vi "BMU诊断标定.vi"(8 "CAN端口":u16(ring), 9 "设备索引号":u16(ring), 10 "CAN卡类型":u32(ring)=21) -> ()   [LabVIEW 2013] (continued)
                                n3887 = property class="Str"(reference=w5555, "Value"="" ("值")) -> ()  [unwired: 1 in, 2 out]
                                }
                                frame "校正时钟" {
                                n3888 = control-ref of="系统时钟"() -> (w5557:refnum<vi>)
                                n3889 = property class="Str"(reference=w5557, "Value"="" ("值")) -> ()  [unwired: 1 in, 2 out]
                                }
                                frame "车牌号" {
                                n3890 = control-ref of="车架(牌)号"() -> (w5559:refnum<vi>)
                                n3891 = property class="Str"(reference=w5559, "Value"="" ("值")) -> ()  [unwired: 1 in, 2 out]
                                }
                                frame "SOH" {
                                n3892 = control-ref of="SOH(%)"() -> (w5562:refnum<vi>)
                                n3893 = property class="DigNum (严格)"(reference=w5562, "Value"=0.0 ("值")) -> ()  [unwired: 1 in, 2 out]
                                }
                                frame "一级故障阀值" {
                                n3894 = local write "一级故障"(T10 {"总电压过高"=0.0, "整组电压不均衡"=0.0, "SOC过高"=0.0, "单体电压过高"=0.0, "总电压过低"=0.0, "温度过高"=0.0, "温度过低"=0.0, "单组电压不均衡"=0.0, "整组温度不均衡"=0.0, "单组温度不均衡"=0.0, "单体电压过低"=0.0, "充电电流过高"=0.0, "放电电流过高"=0.0, "SOC过低"=0.0, "内阻过大"=0.0, "极柱温度过高"=0.0, "SOH过低"=0.0} ("一级故障")) -> ()
                                }
                                frame "二级故障阀值" {
                                n3895 = local write "一级故障 2"(T10 {"总电压过高"=0.0, "整组电压不均衡"=0.0, "SOC过高"=0.0, "单体电压过高"=0.0, "总电压过低"=0.0, "温度过高"=0.0, "温度过低"=0.0, "单组电压不均衡"=0.0, "整组温度不均衡"=0.0, "单组温度不均衡"=0.0, "单体电压过低"=0.0, "充电电流过高"=0.0, "放电电流过高"=0.0, "SOC过低"=0.0, "内阻过大"=0.0, "极柱温度过高"=0.0, "SOH过低"=0.0} ("一级故障")) -> ()
                                }
                                frame "三级故障阀值" {
                                n3896 = local write "一级故障 3"(T10 {"总电压过高"=0.0, "整组电压不均衡"=0.0, "SOC过高"=0.0, "单体电压过高"=0.0, "总电压过低"=0.0, "温度过高"=0.0, "温度过低"=0.0, "单组电压不均衡"=0.0, "整组温度不均衡"=0.0, "单组温度不均衡"=0.0, "单体电压过低"=0.0, "充电电流过高"=0.0, "放电电流过高"=0.0, "SOC过低"=0.0, "内阻过大"=0.0, "极柱温度过高"=0.0, "SOH过低"=0.0} ("一级故障")) -> ()
                                }
                                frame "加热控制参数" {
                                n3897 = local write "加热控制参数"(T11 {"风机开启温度"=0.0, "风机关闭温度"=0.0, "加热开启温度"=0.0, "加热关闭温度"=0.0, "风机开启温差"=0.0, "风机关闭温差"=0.0, "加热关闭温差"=0.0} ("加热控制参数")) -> ()
                                }
                                frame "充电控制参数" {
                                n3898 = local write "一级故障 5"(T12 {"最大允许单体电压"=0.0, "最大允许总电压"=0.0, "最小允许单体电压"=0.0, "最大允许充电电流"=0.0, "最小允许充电电流"=0.0, "最大允许充电温度"=0.0, "最小允许充电温度"=0.0, "电流步长"=0.0} ("一级故障 5")) -> ()
                                }
                                frame "电池信息1" {
                                w5568 = ""
                                w5569 = 0.0 ("电池串联")
                                n3899 = local read "电池信息"() -> (w5571:T13)
                                n3900 = Bundle By Name(cluster=w5571, "电池串联"=w5569, "电池并联"=w5569, "电池包额定容量"=w5569, "电池包额定能量(kWh)"=w5569, "电池包额定总电压"=w5569, "实际容量"=w5569, "电池厂家"=w5568, "电池类型"=w5568, "电池生产日期"=w5568) -> (w5570:T13)
                                n3901 = local write "电池信息"(w5570) -> ()
                                }
                                frame "电池包组号" {
                                n3902 = local read "电池信息"() -> (w5574:T13)
                                n3903 = Bundle By Name(cluster=w5574, "电池包组号"="") -> (w5573:T13)
                                n3904 = local write "电池信息"(w5573) -> ()
                                }
                                frame "充放电安时" {
                                w5575 = 0.0 ("累计充电总安时")
                                n3905 = local read "电池信息"() -> (w5577:T13)
                                n3906 = Bundle By Name(cluster=w5577, "累计充电总安时"=w5575, "累计放电总安时"=w5575) -> (w5576:T13)
                                n3907 = local write "电池信息"(w5576) -> ()
                                }
                                frame "电池充放电次数" {
                                w5578 = 0.0 ("累计充电总安时")
                                n3908 = local read "电池信息"() -> (w5580:T13)
                                n3909 = Bundle By Name(cluster=w5580, "电池充满次数"=w5578, "电池放空次数"=w5578, "电池充电次数"=w5578) -> (w5579:T13)
                                n3910 = local write "电池信息"(w5579) -> ()
                                }
                                }
                              }
                              frame "从板" {
                                n3911 = case shown="\"温度起始值\"" w5581 {
                                frame "假", Default {
                                }
                                frame "电压起始值" {
                                n3912 = for {
                                N: 1 -> [_]
                                tunnel: [""] -> w5586 mode=indexing
                                }
                                n3913 = control-ref of="项目信息 2"() -> (w5582:refnum<vi>)
                                n3914 = call "表格数据输入-8.6.vi"("行数"=u32 0, "列数"=u32 1, "字符串数组"=w5586, "表格引用"=w5582) -> ()  [unwired: 8 in]
                                }
                                frame "通道电压个数" {
                                n3915 = for {
                                N: 5 -> [_]
                                tunnel: [""] -> w5592 mode=indexing
                                }
                                n3916 = control-ref of="项目信息 2"() -> (w5588:refnum<vi>)
                                n3917 = call "表格数据输入-8.6.vi"("行数"=u32 22, "列数"=u32 1, "字符串数组"=w5592, "表格引用"=w5588) -> ()  [unwired: 8 in]
                                }
                                frame "保险位置" {
                                n3918 = for {
                                N: 10 -> [_]
                                tunnel: [""] -> w5598 mode=indexing
                                }
                                n3919 = control-ref of="项目信息 2"() -> (w5594:refnum<vi>)
                                n3920 = call "表格数据输入-8.6.vi"("行数"=u32 2, "列数"=u32 1, "字符串数组"=w5598, "表格引用"=w5594) -> ()  [unwired: 8 in]
                                }
                                frame "温度起始值" {
                                n3921 = for {
                                N: 1 -> [_]
                                tunnel: [""] -> w5604 mode=indexing
                                }
                                n3922 = control-ref of="项目信息 2"() -> (w5600:refnum<vi>)
                                n3923 = call "表格数据输入-8.6.vi"("行数"=u32 1, "列数"=u32 1, "字符串数组"=w5604, "表格引用"=w5600) -> ()  [unwired: 8 in]
                                }
                                frame "加热控制参数" {
                                n3924 = local write "加热控制参数"(T11 {"风机开启温度"=0.0, "风机关闭温度"=0.0, "加热开启温度"=0.0, "加热关闭温度"=0.0, "风机开启温差"=0.0, "风机关闭温差"=0.0, "加热关闭温差"=0.0} ("加热控制参数")) -> ()
                                }
                                frame "一级故障阀值" {
                                n3925 = local write "一级故障 6"(T15 {"电压过高"=0.0, "电压过低"=0.0, "温度过高"=0.0, "温度过低"=0.0, "电压不均衡(V)"=0.0, "温度不均衡"=0.0, "SOC过低"=0.0} ("一级故障 6")) -> ()
                                }
                                frame "二级故障阀值" {
                                n3926 = local write "一级故障 7"(T15 {"电压过高"=0.0, "电压过低"=0.0, "温度过高"=0.0, "温度过低"=0.0, "电压不均衡(V)"=0.0, "温度不均衡"=0.0, "SOC过低"=0.0} ("一级故障 7")) -> ()
                                }
                                frame "三级故障阀值" {
                                n3927 = local write "一级故障 8"(T15 {"电压过高"=0.0, "电压过低"=0.0, "温度过高"=0.0, "温度过低"=0.0, "电压不均衡(V)"=0.0, "温度不均衡"=0.0, "SOC过低"=0.0} ("一级故障 7")) -> ()
                                }
                                frame "均衡参数" {
                                n3928 = local write "均衡参数"(T17 {"充电结束电压(90%)"=0.0, "充电结束电压(91%)"=0.0, "充电结束电压(92%)"=0.0, "充电结束电压(93%)"=0.0, "充电结束电压(94%)"=0.0, "均衡计算-电压高阀值1级"=0.0, "均衡计算-电压高阀值2级"=0.0, "均衡计算-电压低阀值1级"=0.0, "均衡计算-电压低阀值2级"=0.0, "均衡计算-最低电压阀值"=0.0, "均衡停止-最低电压阀值"=0.0, "均衡计算-电压极差阀值"=0.0, "充电结束电压(95%)"=0.0, "充电结束电压(96%)"=0.0, "充电结束电压(97%)"=0.0, "充电结束电压(98%)"=0.0, "充电结束电压(99%)"=0.0, "充电结束电压(100%)"=0.0} ("均衡参数")) -> ()
                                }
                                frame "均衡阀值" {
                                w5611 = sgl 0.0 ("均衡计算-电压高阀值1级")
                                n3929 = local read "均衡参数"() -> (w5612:T17)
                                n3930 = Bundle By Name(cluster=w5612, "均衡计算-电压高阀值1级"=w5611, "均衡计算-电压高阀值2级"=w5611, "均衡计算-电压低阀值1级"=w5611, "均衡计算-电压低阀值2级"=w5611, "均衡计算-最低电压阀值"=w5611, "均衡停止-最低电压阀值"=w5611, "均衡计算-电压极差阀值"=w5611) -> (w5613:T17)
                                n3931 = local write "均衡参数"(w5613) -> ()
                                }
                                frame "充电结束电压" {
                                w5614 = sgl 0.0 ("均衡计算-电压高阀值1级")
                                n3932 = local read "均衡参数"() -> (w5615:T17)
                                n3933 = Bundle By Name(cluster=w5615, "充电结束电压(90%)"=w5614, "充电结束电压(91%)"=w5614, "充电结束电压(92%)"=w5614, "充电结束电压(93%)"=w5614, "充电结束电压(94%)"=w5614, "充电结束电压(95%)"=w5614, "充电结束电压(96%)"=w5614, "充电结束电压(97%)"=w5614, "充电结束电压(98%)"=w5614, "充电结束电压(99%)"=w5614, "充电结束电压(100%)"=w5614) -> (w5616:T17)
                                n3934 = local write "均衡参数"(w5616) -> ()
                                }
                                }
                              }
                            }
                          }
                          frame #1 {
                            w5617 = FALSE ("流控帧")
                            w5618 = TRUE ("流控帧 2")
                            n3935 = global write "EV05全局变量1.vi" "写入超时"(w5617) -> ()
                            n3936 = global write "EV05全局变量1.vi" "流控帧"(w5617) -> ()
                            n3937 = local write "写?"(w5617) -> ()
                            n3938 = local write "消除"(w5618) -> ()
                            n3939 = local write "控制1"(w5618) -> ()
                            n3940 = global write "EV05全局变量1.vi" "流控帧 2"(w5618) -> ()
                          }
                          frame #2 {
                            n3941 = Wait Until Next ms Multiple(millisecond multiple=u32 300 ("毫秒倍数")) -> ()  [unwired: 1 out]
                          }
                          frame #3 {
                            n3942 = local read "设备索引号"() -> (w5621:u16)
                            n3943 = local read "CAN卡类型"() -> (w5622:u32)
                            n3944 = local read "CAN端口"() -> (w5620:u16)
                            n3945 = local write "命令序号"(w5625) -> ()
                            n3946 = stacked-sequence {
                              tunnel: w5626 -> [_ w5633]
                              tunnel: w5625 -> [_ w5632]
                              tunnel: w5624 -> [_ w5631]
                              tunnel: w5623 -> [_ w5630]
                              tunnel: w5622 -> [_ w5629]
                              tunnel: w5621 -> [_ w5628]
                              tunnel: w5620 -> [_ w5627]
                              frame #0 {
                              }
                              frame #1 {
                                n3947 = call "多帧发送机制(EV05).vi"("can卡类型"=w5629, "设备索引号"=w5628, "CAN端口"=w5627, "命令"=w5633, "板号"=w5631, "命令序号"=w5632, "输入数据"=w5630) -> ()  [unwired: 1 in, 12 out]
                              }
                            }
                          }
                          frame #4 {
                            n3948 = while {
                              tunnel: [w5638] -> w5635
                              tunnel: [w5637] -> w5634
                              i -> [w5641]
                              stop <- w5638 stop-if-true
                              n3949 = local read "强制终止读写标记"() -> (w5636:bool)
                              n3950 = global read "EV05全局变量1.vi" "写入超时"() -> (w5637:bool)
                              n3951 = Greater Or Equal?(x=w5641, y=20) -> (x >= y?=w5639:bool)
                              n3952 = Compound Arithmetic op=OR(w5636, w5637, w5639) -> (w5638:bool)
                              n3953 = Wait Until Next ms Multiple(millisecond multiple=u32 100 ("毫秒倍数")) -> ()  [unwired: 1 out]
                            }
                          }
                          frame #5 {
                            n3954 = case shown="假" w5650 {
                              tunnel: w5649 -> [w5661 _]
                              tunnel: [w5656 w5673] -> w5648
                              tunnel: w5647 -> [w5655 _]
                              tunnel: w5646 -> [w5654 w5673]
                              tunnel: [w5653 w5672] -> w5643
                              tunnel: w5645 -> [w5652 _]
                              tunnel: w5644 -> [w5651 w5672]
                              frame False {
                                n3955 = local read "重试次数"() -> (w5660:u8)
                                n3956 = Increment(x=w5660) -> (x+1=w5659:u8)
                                n3957 = Greater Or Equal?(x=w5659, y=u8 4) -> (x >= y?=w5658:bool)
                                n3958 = local write "重试次数"(w5659) -> ()
                                n3959 = case shown="真" w5658 {
                                tunnel: w5661 -> [_ w5666]
                                tunnel: [w5663 w5665] -> w5656
                                tunnel: w5655 -> [w5663 _]
                                tunnel: w5654 -> [_ w5665]
                                tunnel: [w5662 w5664] -> w5653
                                tunnel: w5652 -> [w5662 _]
                                tunnel: w5651 -> [_ w5664]
                                frame False {
                                }
                                frame True {
                                n3960 = control-ref of="结果"() -> (w5668:refnum<vi>)
                                n3961 = Concatenate Strings(w5666, "     读取失败" ("字符串")) -> (w5670:string)
                                n3962 = Build Array(w5670) -> (w5667:string[])
                                n3963 = call "表格编辑.vi"("新元素/子数组"=w5667, "活动单元格:单元格背景色"=u32 16740749, "MCListbox引用句柄"=w5668) -> ()  [unwired: 9 out]
                                }
                                }
                              }
                              frame True {
                              }
                            }
                          }
                          frame #6 {
                            n3964 = And(x=w5675, y=w5677) -> (x .and. y?=w5676:bool)
                            n3965 = case shown="真" w5676 {
                              frame False {
                              }
                              frame True {
                                n3966 = local write "强制终止读写标记"(FALSE ("强制停止")) -> ()
                                n3967 = control-ref of="结果"() -> (w5680:refnum<vi>)
                                n3968 = Concatenate Strings("读取完成" ("字符串")) -> (w5682:string)
                                n3969 = Build Array(w5682) -> (w5679:string[])
                                n3970 = call "表格编辑.vi"("新元素/子数组"=w5679, "活动单元格:单元格背景色"=u32 21937, "MCListbox引用句柄"=w5680) -> ()  [unwired: 9 out]
                              }
                            }
                            n3971 = Wait (ms)(milliseconds to wait=u32 50 ("等待时间（毫秒）")) -> ()  [unwired: 1 out]
                          }
                        }
                      }
                    }
                  }
                  n3972 = local read "强制终止读写标记"() -> (w5448:bool)
                  n3973 = Or(x=w5448, y=w5447) -> (x .or. y?=w5445:bool)
                }
              }
            }
            frame #2 {
              n3974 = case shown="假" w5767 {
                tunnel: w5768 -> [w5769 _]
                frame False {
                  n3975 = case shown="\"主板\", 默认" w5769 {
                    frame "主板", Default {
                      n3976 = global read "读配置文件全局.vi" "电池额定实际容量判定"() -> (w5783:bool)
                      n3977 = global read "读配置文件全局.vi" "电池充放电次数判定"() -> (w5772:bool)
                      n3978 = global read "读配置文件全局.vi" "加热控制参数判定"() -> (w5770:bool)
                      n3979 = global read "读配置文件全局.vi" "配置文件版本判定"() -> (w5782:bool)
                      n3980 = global read "读配置文件全局.vi" "充电控制参数判定"() -> (w5776:bool)
                      n3981 = global read "读配置文件全局.vi" "通道电压数判定"() -> (w5788:bool)
                      n3982 = global read "读配置文件全局.vi" "电压起始值判定"() -> (w5787:bool)
                      n3983 = global read "读配置文件全局.vi" "温度起始值判定"() -> (w5785:bool)
                      n3984 = global read "读配置文件全局.vi" "充放电安时判定"() -> (w5774:bool)
                      n3985 = global read "读配置文件全局.vi" "电池包组号判定"() -> (w5773:bool)
                      n3986 = global read "读配置文件全局.vi" "电池信息1判定"() -> (w5775:bool)
                      n3987 = global read "读配置文件全局.vi" "从板个数判定"() -> (w5791:bool)
                      n3988 = global read "读配置文件全局.vi" "产品编号判定"() -> (w5790:bool)
                      n3989 = global read "读配置文件全局.vi" "电压个数判定"() -> (w5789:bool)
                      n3990 = global read "读配置文件全局.vi" "温度个数判定"() -> (w5786:bool)
                      n3991 = global read "读配置文件全局.vi" "保险位置判定"() -> (w5784:bool)
                      n3992 = global read "读配置文件全局.vi" "一级故障判定"() -> (w5779:bool)
                      n3993 = global read "读配置文件全局.vi" "二级故障判定"() -> (w5778:bool)
                      n3994 = global read "读配置文件全局.vi" "三级故障判定"() -> (w5777:bool)
                      n3995 = global read "读配置文件全局.vi" "车牌号判定"() -> (w5781:bool)
                      n3996 = global read "读配置文件全局.vi" "SOH判定"() -> (w5780:bool)
                      n3997 = Build Array(w5791, w5790, w5789, w5788, w5787, w5786, w5785, w5784, w5783, w5782, w5781, w5780, w5779, w5778, w5777, w5776, w5775, w5774, w5773, w5772, w5770) -> (w5771:bool[])
                      n3998 = And Array Elements(Boolean array=w5771) -> (logical AND=w5792:bool)
                      n3999 = disable-structure shown="禁用" {
                        frame Disabled {
                          n4000 = global read "读配置文件全局.vi" "SOC判定"() -> ()  [unwired: 1 out]
                        }
                        frame Enabled {
                        }
                      }
                      n4001 = case shown="假" w5792 {
                        tunnel: w5771 -> [_ w5797]
                        frame True {
                          n4002 = control-ref of="结果"() -> (w5795:refnum<vi>)
                          n4003 = Build Array("全部判定成功!!!!!!!!") -> (w5796:string[])
                          n4004 = call "表格编辑.vi"("新元素/子数组"=w5796, "活动单元格:单元格背景色"=u32 6618880, "MCListbox引用句柄"=w5795) -> ()  [unwired: 9 out]
                        }
                        frame False {
                          n4005 = stacked-sequence {
                            tunnel: w5797 -> [_ w5802]
                            frame #0 {
                              n4006 = control-ref of="结果"() -> (w5800:refnum<vi>)
                              n4007 = Build Array("全部判定失败!!!!!") -> (w5801:string[])
                              n4008 = call "表格编辑.vi"("新元素/子数组"=w5801, "活动单元格:单元格背景色"=u32 16711680, "MCListbox引用句柄"=w5800) -> ()  [unwired: 9 out]
                            }
                            frame #1 {
                              n4009 = for {
                                tunnel: w5802 -> [w5804] mode=indexing
                                i -> [w5803]
                                n4010 = case shown="20" w5803 {
                                tunnel: w5804 -> [w5805 w5810 w5815 w5820 w5825 w5830 w5835 w5840 w5845 w5850 w5855 w5860 w5865 w5870 w5875 w5880 w5885 w5890 w5895 w5900 w5905 _]
                                frame 0 {
                                n4011 = case shown="假" w5805 {
                                frame False {
                                n4012 = control-ref of="结果"() -> (w5808:refnum<vi>)
                                n4013 = Build Array("从板个数判定失败!") -> (w5809:string[])
                                n4014 = call "表格编辑.vi"("新元素/子数组"=w5809, "活动单元格:单元格背景色"=u32 16711680, "MCListbox引用句柄"=w5808) -> ()  [unwired: 9 out]
                                }
                                frame True {
                                }
                                }
                                }
                                frame 1 {
                                n4015 = case shown="假" w5810 {
                                frame False {
                                n4016 = control-ref of="结果"() -> (w5813:refnum<vi>)
                                n4017 = Build Array("产品编号判定失败!") -> (w5814:string[])
                                n4018 = call "表格编辑.vi"("新元素/子数组"=w5814, "活动单元格:单元格背景色"=u32 16711680, "MCListbox引用句柄"=w5813) -> ()  [unwired: 9 out]
                                }
                                frame True {
                                }
                                }
                                }
                                frame 2 {
                                n4019 = case shown="假" w5815 {
                                frame False {
                                n4020 = control-ref of="结果"() -> (w5818:refnum<vi>)
                                n4021 = Build Array("电压个数判定失败!") -> (w5819:string[])
                                n4022 = call "表格编辑.vi"("新元素/子数组"=w5819, "活动单元格:单元格背景色"=u32 16711680, "MCListbox引用句柄"=w5818) -> ()  [unwired: 9 out]
                                }
                                frame True {
                                }
                                }
                                }
                                frame 3 {
                                n4023 = case shown="假" w5820 {
                                frame False {
                                n4024 = control-ref of="结果"() -> (w5823:refnum<vi>)
                                n4025 = Build Array("通道电压数判定失败!") -> (w5824:string[])
                                n4026 = call "表格编辑.vi"("新元素/子数组"=w5824, "活动单元格:单元格背景色"=u32 16711680, "MCListbox引用句柄"=w5823) -> ()  [unwired: 9 out]
                                }
                                frame True {
                                }
                                }
                                }
                                frame 4 {
                                n4027 = case shown="假" w5825 {
                                frame False {
                                n4028 = control-ref of="结果"() -> (w5828:refnum<vi>)
                                n4029 = Build Array("电压起始值判定失败!") -> (w5829:string[])
                                n4030 = call "表格编辑.vi"("新元素/子数组"=w5829, "活动单元格:单元格背景色"=u32 16711680, "MCListbox引用句柄"=w5828) -> ()  [unwired: 9 out]
                                }
                                frame True {
                                }
                                }
                                }
                                frame 5 {
                                n4031 = case shown="假" w5830 {
                                frame False {
                                n4032 = control-ref of="结果"() -> (w5833:refnum<vi>)
                                n4033 = Build Array("温度个数判定失败!") -> (w5834:string[])
                                n4034 = call "表格编辑.vi"("新元素/子数组"=w5834, "活动单元格:单元格背景色"=u32 16711680, "MCListbox引用句柄"=w5833) -> ()  [unwired: 9 out]
                                }
                                frame True {
                                }
                                }
                                }
                                frame 6 {
                                n4035 = case shown="假" w5835 {
                                frame False {
                                n4036 = control-ref of="结果"() -> (w5838:refnum<vi>)
                                n4037 = Build Array("温度起始值判定失败!") -> (w5839:string[])
                                n4038 = call "表格编辑.vi"("新元素/子数组"=w5839, "活动单元格:单元格背景色"=u32 16711680, "MCListbox引用句柄"=w5838) -> ()  [unwired: 9 out]
                                }
                                frame True {
                                }
                                }
                                }
                                frame 7 {
                                n4039 = case shown="假" w5840 {
                                frame False {
                                n4040 = control-ref of="结果"() -> (w5843:refnum<vi>)
                                n4041 = Build Array("保险位置判定失败!") -> (w5844:string[])
                                n4042 = call "表格编辑.vi"("新元素/子数组"=w5844, "活动单元格:单元格背景色"=u32 16711680, "MCListbox引用句柄"=w5843) -> ()  [unwired: 9 out]
                                }
                                frame True {
                                }
                                }
                                }
                                frame 8 {
                                n4043 = case shown="假" w5845 {
                                frame False {
                                n4044 = control-ref of="结果"() -> (w5848:refnum<vi>)
                                n4045 = Build Array("电池额定实际容量判定失败!") -> (w5849:string[])
                                n4046 = call "表格编辑.vi"("新元素/子数组"=w5849, "活动单元格:单元格背景色"=u32 16711680, "MCListbox引用句柄"=w5848) -> ()  [unwired: 9 out]
                                }
                                frame True {
                                }
                                }
                                }
                                frame 9 {
                                n4047 = case shown="假" w5850 {
                                frame False {
                                n4048 = control-ref of="结果"() -> (w5853:refnum<vi>)
                                n4049 = Build Array("配置文件版本判定失败!") -> (w5854:string[])
                                n4050 = call "表格编辑.vi"("新元素/子数组"=w5854, "活动单元格:单元格背景色"=u32 16711680, "MCListbox引用句柄"=w5853) -> ()  [unwired: 9 out]
                                }
                                frame True {
                                }
                                }
                                }
                                frame 10 {
                                n4051 = case shown="假" w5855 {
                                frame False {
                                n4052 = control-ref of="结果"() -> (w5858:refnum<vi>)
                                n4053 = Build Array("车牌号判定失败!") -> (w5859:string[])
                                n4054 = call "表格编辑.vi"("新元素/子数组"=w5859, "活动单元格:单元格背景色"=u32 16711680, "MCListbox引用句柄"=w5858) -> ()  [unwired: 9 out]
                                }
                                frame True {
                                }
                                }
                                }
                                frame 11 {
                                n4055 = case shown="假" w5860 {
                                frame False {
                                n4056 = control-ref of="结果"() -> (w5863:refnum<vi>)
                                n4057 = Build Array("SOH判定失败!") -> (w5864:string[])
                                n4058 = call "表格编辑.vi"("新元素/子数组"=w5864, "活动单元格:单元格背景色"=u32 16711680, "MCListbox引用句柄"=w5863) -> ()  [unwired: 9 out]
                                }
                                frame True {
                                }
                                }
                                }
                                frame 12 {
                                n4059 = case shown="假" w5865 {
                                frame False {
                                n4060 = control-ref of="结果"() -> (w5868:refnum<vi>)
                                n4061 = Build Array("一级故障阀值判定失败!") -> (w5869:string[])
                                n4062 = call "表格编辑.vi"("新元素/子数组"=w5869, "活动单元格:单元格背景色"=u32 16711680, "MCListbox引用句柄"=w5868) -> ()  [unwired: 9 out]
                                }
                                frame True {
                                }
                                }
                                }
                                frame 13 {
                                n4063 = case shown="假" w5870 {
                                frame False {
                                n4064 = control-ref of="结果"() -> (w5873:refnum<vi>)
                                n4065 = Build Array("二级故障阀值判定失败!") -> (w5874:string[])
                                n4066 = call "表格编辑.vi"("新元素/子数组"=w5874, "活动单元格:单元格背景色"=u32 16711680, "MCListbox引用句柄"=w5873) -> ()  [unwired: 9 out]
                                }
                                frame True {
                                }
                                }
                                }
                                frame 14 {
                                n4067 = case shown="假" w5875 {
                                frame False {
                                n4068 = control-ref of="结果"() -> (w5878:refnum<vi>)
                                n4069 = Build Array("三级故障阀值判定失败!") -> (w5879:string[])
                                n4070 = call "表格编辑.vi"("新元素/子数组"=w5879, "活动单元格:单元格背景色"=u32 16711680, "MCListbox引用句柄"=w5878) -> ()  [unwired: 9 out]
                                }
                                frame True {
                                }
                                }
                                }
                                frame 15 {
                                n4071 = case shown="假" w5880 {
                                frame False {
                                n4072 = control-ref of="结果"() -> (w5883:refnum<vi>)
                                n4073 = Build Array("充电控制参数判定失败!") -> (w5884:string[])
                                n4074 = call "表格编辑.vi"("新元素/子数组"=w5884, "活动单元格:单元格背景色"=u32 16711680, "MCListbox引用句柄"=w5883) -> ()  [unwired: 9 out]
                                }
                                frame True {
                                }
                                }
                                }
                                frame 16 {
                                n4075 = case shown="假" w5885 {
                                frame False {
                                n4076 = control-ref of="结果"() -> (w5888:refnum<vi>)
                                n4077 = Build Array("电池信息1判定失败!") -> (w5889:string[])
                                n4078 = call "表格编辑.vi"("新元素/子数组"=w5889, "活动单元格:单元格背景色"=u32 16711680, "MCListbox引用句柄"=w5888) -> ()  [unwired: 9 out]
                                }
                                frame True {
                                }
                                }
                                }
                                frame 17 {
                                n4079 = case shown="假" w5890 {
                                frame False {
                                n4080 = control-ref of="结果"() -> (w5893:refnum<vi>)
                                n4081 = Build Array("充放电安时判定失败!") -> (w5894:string[])
                                n4082 = call "表格编辑.vi"("新元素/子数组"=w5894, "活动单元格:单元格背景色"=u32 16711680, "MCListbox引用句柄"=w5893) -> ()  [unwired: 9 out]
                                }
                                frame True {
                                }
                                }
                                }
                                frame 18 {
                                n4083 = case shown="假" w5895 {
                                frame False {
                                n4084 = control-ref of="结果"() -> (w5898:refnum<vi>)
                                n4085 = Build Array("电池包组号判定失败!") -> (w5899:string[])
                                n4086 = call "表格编辑.vi"("新元素/子数组"=w5899, "活动单元格:单元格背景色"=u32 16711680, "MCListbox引用句柄"=w5898) -> ()  [unwired: 9 out]
                                }
                                frame True {
                                }
                                }
                                }
                                frame 19 {
                                n4087 = case shown="假" w5900 {
                                frame False {
                                n4088 = control-ref of="结果"() -> (w5903:refnum<vi>)
                                n4089 = Build Array("电池充放电次数判定失败!") -> (w5904:string[])
                                n4090 = call "表格编辑.vi"("新元素/子数组"=w5904, "活动单元格:单元格背景色"=u32 16711680, "MCListbox引用句柄"=w5903) -> ()  [unwired: 9 out]
                                }
                                frame True {
                                }
                                }
                                }
                                frame 20 {
                                n4091 = case shown="假" w5905 {
                                frame False {
                                n4092 = control-ref of="结果"() -> (w5908:refnum<vi>)
                                n4093 = Build Array("加热控制参数判定失败!") -> (w5909:string[])
                                n4094 = call "表格编辑.vi"("新元素/子数组"=w5909, "活动单元格:单元格背景色"=u32 16711680, "MCListbox引用句柄"=w5908) -> ()  [unwired: 9 out]
                                }
                                frame True {
                                }
                                }
                                }
                                frame 99, Default {
                                }
                                }
                              }
                            }
                          }
                        }
                      }
                    }
                    frame "从板" {
                      n4095 = global read "读配置文件全局2.vi" "电压起始值判定"() -> (w5918:bool)
                      n4096 = global read "读配置文件全局2.vi" "温度起始值判定"() -> (w5915:bool)
                      n4097 = global read "读配置文件全局2.vi" "加热控制参数判定"() -> (w5910:bool)
                      n4098 = global read "读配置文件全局2.vi" "通道电压判定"() -> (w5917:bool)
                      n4099 = global read "读配置文件全局2.vi" "保险位置判定"() -> (w5916:bool)
                      n4100 = global read "读配置文件全局2.vi" "一级故障判定"() -> (w5913:bool)
                      n4101 = global read "读配置文件全局2.vi" "二级故障判定"() -> (w5912:bool)
                      n4102 = global read "读配置文件全局2.vi" "三级故障判定"() -> (w5911:bool)
                      n4103 = global read "读配置文件全局2.vi" "从板号判定"() -> (w5919:bool)
                      n4104 = Build Array(w5919, w5918, w5917, w5916, w5915, w5913, w5912, w5911, w5910) -> (w5914:bool[])
                      n4105 = And Array Elements(Boolean array=w5914) -> (logical AND=w5920:bool)
                      n4106 = case shown="假" w5920 {
                        tunnel: w5914 -> [_ w5925]
                        frame True {
                          n4107 = control-ref of="结果"() -> (w5923:refnum<vi>)
                          n4108 = Build Array("读取判定成功!!!!!!!!") -> (w5924:string[])
                          n4109 = call "表格编辑.vi"("新元素/子数组"=w5924, "活动单元格:单元格背景色"=u32 6618880, "MCListbox引用句柄"=w5923) -> ()  [unwired: 9 out]
                        }
                        frame False {
                          n4110 = stacked-sequence {
                            tunnel: w5925 -> [_ w5930]
                            frame #0 {
                              n4111 = control-ref of="结果"() -> (w5928:refnum<vi>)
                              n4112 = Build Array("读取判定失败!!!!!") -> (w5929:string[])
                              n4113 = call "表格编辑.vi"("新元素/子数组"=w5929, "活动单元格:单元格背景色"=u32 16711680, "MCListbox引用句柄"=w5928) -> ()  [unwired: 9 out]
                            }
                            frame #1 {
                              n4114 = for {
                                tunnel: w5930 -> [w5931] mode=indexing
                                i -> [w5932]
                                n4115 = case shown="0" w5932 {
                                tunnel: w5931 -> [w5933 w5938 w5943 w5948 w5953 w5958 w5963 w5968 w5973 _]
                                frame 0 {
                                n4116 = case shown="假" w5933 {
                                frame False {
                                n4117 = control-ref of="结果"() -> (w5936:refnum<vi>)
                                n4118 = Build Array("从板号判定失败!") -> (w5937:string[])
                                n4119 = call "表格编辑.vi"("新元素/子数组"=w5937, "活动单元格:单元格背景色"=u32 16711680, "MCListbox引用句柄"=w5936) -> ()  [unwired: 9 out]
                                }
                                frame True {
                                }
                                }
                                }
                                frame 1 {
                                n4120 = case shown="假" w5938 {
                                frame False {
                                n4121 = control-ref of="结果"() -> (w5941:refnum<vi>)
                                n4122 = Build Array("电压起始值判定失败!") -> (w5942:string[])
                                n4123 = call "表格编辑.vi"("新元素/子数组"=w5942, "活动单元格:单元格背景色"=u32 16711680, "MCListbox引用句柄"=w5941) -> ()  [unwired: 9 out]
                                }
                                frame True {
                                }
                                }
                                }
                                frame 2 {
                                n4124 = case shown="假" w5943 {
                                frame False {
                                n4125 = control-ref of="结果"() -> (w5946:refnum<vi>)
                                n4126 = Build Array("通道电压节数判定失败!") -> (w5947:string[])
                                n4127 = call "表格编辑.vi"("新元素/子数组"=w5947, "活动单元格:单元格背景色"=u32 16711680, "MCListbox引用句柄"=w5946) -> ()  [unwired: 9 out]
                                }
                                frame True {
                                }
                                }
                                }
                                frame 3 {
                                n4128 = case shown="假" w5948 {
                                frame False {
                                n4129 = control-ref of="结果"() -> (w5951:refnum<vi>)
                                n4130 = Build Array("保险位置判定失败!") -> (w5952:string[])
                                n4131 = call "表格编辑.vi"("新元素/子数组"=w5952, "活动单元格:单元格背景色"=u32 16711680, "MCListbox引用句柄"=w5951) -> ()  [unwired: 9 out]
                                }
                                frame True {
                                }
                                }
                                }
                                frame 4 {
                                n4132 = case shown="假" w5953 {
                                frame False {
                                n4133 = control-ref of="结果"() -> (w5956:refnum<vi>)
                                n4134 = Build Array("温度起始值判定失败!") -> (w5957:string[])
                                n4135 = call "表格编辑.vi"("新元素/子数组"=w5957, "活动单元格:单元格背景色"=u32 16711680, "MCListbox引用句柄"=w5956) -> ()  [unwired: 9 out]
                                }
                                frame True {
                                }
                                }
                                }
                                frame 5 {
                                n4136 = case shown="假" w5958 {
                                frame False {
                                n4137 = control-ref of="结果"() -> (w5961:refnum<vi>)
                                n4138 = Build Array("一级故障判定失败!") -> (w5962:string[])
                                n4139 = call "表格编辑.vi"("新元素/子数组"=w5962, "活动单元格:单元格背景色"=u32 16711680, "MCListbox引用句柄"=w5961) -> ()  [unwired: 9 out]
                                }
                                frame True {
                                }
                                }
                                }
                                frame 6 {
                                n4140 = case shown="假" w5963 {
                                frame False {
                                n4141 = control-ref of="结果"() -> (w5966:refnum<vi>)
                                n4142 = Build Array("二级故障判定失败!") -> (w5967:string[])
                                n4143 = call "表格编辑.vi"("新元素/子数组"=w5967, "活动单元格:单元格背景色"=u32 16711680, "MCListbox引用句柄"=w5966) -> ()  [unwired: 9 out]
                                }
                                frame True {
                                }
                                }
                                }
                                frame 7 {
                                n4144 = case shown="假" w5968 {
                                frame False {
                                n4145 = control-ref of="结果"() -> (w5971:refnum<vi>)
                                n4146 = Build Array("三级故障判定失败!") -> (w5972:string[])
                                n4147 = call "表格编辑.vi"("新元素/子数组"=w5972, "活动单元格:单元格背景色"=u32 16711680, "MCListbox引用句柄"=w5971) -> ()  [unwired: 9 out]
                                }
                                frame True {
                                }
                                }
                                }
                                frame 8 {
                                n4148 = case shown="假" w5973 {
                                frame False {
                                n4149 = control-ref of="结果"() -> (w5976:refnum<vi>)
                                n4150 = Build Array("加热控制参数判定失败!") -> (w5977:string[])
                                n4151 = call "表格编辑.vi"("新元素/子数组"=w5977, "活动单元格:单元格背景色"=u32 16711680, "MCListbox引用句柄"=w5976) -> ()  [unwired: 9 out]
                                }
                                frame True {
                                }
                                }
                                }
                                frame 99, Default {
                                }
                                }
                              }
                            }
                          }
                        }
                      }
                      n4152 = disable-structure shown="禁用" {
                        frame Disabled {
                          n4153 = global read "读配置文件全局.vi" "SOC判定"() -> ()  [unwired: 1 out]
                        }
                        frame Enabled {
                        }
                      }
                    }
                  }
                }
                frame True {
                }
              }
            }
          }
          n4154 = stacked-sequence {
            tunnel: w5210 -> [_]
            frame #0 {
              n4155 = local write "强制终止读写标记"(FALSE ("强制停止")) -> ()
            }
          }
          "重试次数" <- u8 0 ("重试次数")
        }
        frame "开启均衡" {
          n4156 = local read "从板板号"() -> (w5978:u8)
          n4157 = stacked-sequence {
            tunnel: 133 -> [_ w6004 _ _]
            tunnel: w5978 -> [_ _ _ _]
            frame #0 {
              w5988 = u8 0 items=["Normal", "Listen Only"] ("工作方式")
              w5987 = u8 1 items=["Dual Filter", "Single Filter"] ("滤波方式")
              n4158 = global write "EV05全局变量1.vi" "读取超时"(FALSE ("读取超时")) -> ()
              n4159 = global write "EV05全局变量1.vi" "流控帧 2"(TRUE ("流控帧 2")) -> ()
              n4160 = local write "写?"(TRUE ("写?")) -> ()
              n4161 = local read "设备索引号"() -> (w5983:u16)
              n4162 = local read "CAN卡类型"() -> (w5982:u32)
              n4163 = local read "CAN端口"() -> (w5984:u16)
              n4164 = local write "控制1"(TRUE ("控制1")) -> ()
              n4165 = local write "消除"(TRUE ("消除")) -> ()
              n4166 = global write "EV05全局变量1.vi" "流控帧"(FALSE ("流控帧")) -> ()
              n4167 = call "CAN_Init-8.6.vi"("CAN卡类型"=w5982, "设备索引号"=w5983, "CAN端口"=w5984, "操作类型"=enum16{"初始化CAN", "关闭CAN"}."初始化CAN", "滤波方式"=w5987, "Accept Code"=u32 606601216, "簇"=T23 {"打开CAN"=FALSE, "初始化CAN"=TRUE, "开始CAN"=TRUE, "重启"=FALSE, "关闭CAN"=FALSE}, "Mask Code"=u32 524287 ("Accept Code"), "工作方式"=w5988, "是否滤波"=TRUE, "滤波选择"=T22 {"fiter_mode"=1, "fiter_endid"=75825152, "fiter_startid"=75890687}) -> ()  [unwired: 3 in, 6 out]
              n4168 = Wait Until Next ms Multiple(millisecond multiple=u32 20 ("毫秒倍数")) -> ()  [unwired: 1 out]
            }
            frame #1 {
              n4169 = local write "命令"(w6004) -> ()
              n4170 = call "ID组合.vi"("SA(4)"=0 ("PDU(1)"), "PS(3)"=63 ("PDU(1)"), "PF(2)"=w6004, "PDU(1)"=4) -> ("ID"=w6003:i32)  [unwired: 7 out]
              n4171 = local read "均衡类型选择"() -> (w6000:enum16{"放电均衡", "充电均衡", "充放电均衡"})
              n4172 = local read "设备索引号"() -> (w6009:u16)
              n4173 = local read "CAN卡类型"() -> (w6010:u32)
              n4174 = local read "CAN端口"() -> (w6008:u16)
              n4175 = local write "命令序号"(2) -> ()
              n4176 = Add(x=w6000, y=1) -> (x+y=w5998:i32)
              n4177 = Build Array(2, 2, w5998) -> (w6011:i32[])
              n4178 = call "transmit-8.6.vi"("can卡类型"=w6010, "设备索引号"=w6009, "CAN端口"=w6008, "ID"=w6003, "SendType"=u8 0, "Data"=w6011) -> ()  [unwired: 3 in, 11 out]
            }
            frame #2 {
              n4179 = Wait Until Next ms Multiple(millisecond multiple=u32 1000 ("毫秒倍数")) -> ()  [unwired: 1 out]
            }
            frame #3 {
              w6019 = u8 0 items=["Normal", "Listen Only"] ("工作方式")
              w6020 = u8 1 items=["Dual Filter", "Single Filter"] ("滤波方式")
              n4180 = global write "EV05全局变量1.vi" "流控帧 2"(FALSE ("流控帧 2")) -> ()
              n4181 = local read "CAN卡类型"() -> (w6025:u32)
              n4182 = local read "设备索引号"() -> (w6024:u16)
              n4183 = local read "CAN端口"() -> (w6023:u16)
              n4184 = local write "控制1"(FALSE ("控制1")) -> ()
              n4185 = local write "消除"(FALSE ("消除")) -> ()
              n4186 = call <vilib>:"Unset Busy.vi"() -> ()  [unwired: 2 in, 10 out]
              n4187 = call "CAN_Init-8.6.vi"("CAN卡类型"=w6025, "设备索引号"=w6024, "CAN端口"=w6023, "操作类型"=enum16{"初始化CAN", "关闭CAN"}."初始化CAN", "滤波方式"=w6020, "Accept Code"=u32 3221225472, "簇"=T23 {"打开CAN"=FALSE, "初始化CAN"=TRUE, "开始CAN"=TRUE, "重启"=FALSE, "关闭CAN"=FALSE}, "Mask Code"=u32 1073741823 ("Accept Code"), "工作方式"=w6019, "是否滤波"=TRUE, "滤波选择"=T22 {"fiter_mode"=1, "fiter_endid"=402653184, "fiter_startid"=419430399}) -> ()  [unwired: 3 in, 6 out]
            }
          }
        }
        frame "关闭均衡" {
          n4188 = local read "从板板号"() -> (w6029:u8)
          n4189 = stacked-sequence {
            tunnel: 133 -> [_ w6053 _ _]
            tunnel: w6029 -> [_ _ _ _]
            frame #0 {
              w6039 = u8 0 items=["Normal", "Listen Only"] ("工作方式")
              w6038 = u8 1 items=["Dual Filter", "Single Filter"] ("滤波方式")
              n4190 = global write "EV05全局变量1.vi" "读取超时"(FALSE ("读取超时")) -> ()
              n4191 = global write "EV05全局变量1.vi" "流控帧 2"(TRUE ("流控帧 2")) -> ()
              n4192 = local write "写?"(TRUE ("写?")) -> ()
              n4193 = local read "设备索引号"() -> (w6034:u16)
              n4194 = local read "CAN卡类型"() -> (w6033:u32)
              n4195 = local read "CAN端口"() -> (w6035:u16)
              n4196 = local write "控制1"(TRUE ("控制1")) -> ()
              n4197 = global write "EV05全局变量1.vi" "流控帧"(FALSE ("流控帧")) -> ()
              n4198 = local write "消除"(TRUE ("消除")) -> ()
              n4199 = call "CAN_Init-8.6.vi"("CAN卡类型"=w6033, "设备索引号"=w6034, "CAN端口"=w6035, "操作类型"=enum16{"初始化CAN", "关闭CAN"}."初始化CAN", "滤波方式"=w6038, "Accept Code"=u32 606601216, "簇"=T23 {"打开CAN"=FALSE, "初始化CAN"=TRUE, "开始CAN"=TRUE, "重启"=FALSE, "关闭CAN"=FALSE}, "Mask Code"=u32 524287 ("Accept Code"), "工作方式"=w6039, "是否滤波"=TRUE, "滤波选择"=T22 {"fiter_mode"=1, "fiter_endid"=75825152, "fiter_startid"=75890687}) -> ()  [unwired: 3 in, 6 out]
              n4200 = Wait Until Next ms Multiple(millisecond multiple=u32 20 ("毫秒倍数")) -> ()  [unwired: 1 out]
            }
            frame #1 {
              n4201 = local write "命令"(w6053) -> ()
              n4202 = call "ID组合.vi"("SA(4)"=0 ("PDU(1)"), "PS(3)"=63 ("PDU(1)"), "PF(2)"=w6053, "PDU(1)"=4) -> ("ID"=w6052:i32)  [unwired: 7 out]
              n4203 = local read "均衡类型选择"() -> (w6063:enum16{"放电均衡", "充电均衡", "充放电均衡"})
              n4204 = local write "命令序号"(3) -> ()
              n4205 = local read "设备索引号"() -> (w6058:u16)
              n4206 = local read "CAN卡类型"() -> (w6059:u32)
              n4207 = local read "CAN端口"() -> (w6057:u16)
              n4208 = Add(x=w6063, y=1) -> (x+y=w6061:i32)
              n4209 = Build Array(2, 3, w6061) -> (w6060:i32[])
              n4210 = call "transmit-8.6.vi"("can卡类型"=w6059, "设备索引号"=w6058, "CAN端口"=w6057, "ID"=w6052, "SendType"=u8 0, "Data"=w6060) -> ()  [unwired: 3 in, 11 out]
            }
            frame #2 {
              n4211 = Wait Until Next ms Multiple(millisecond multiple=u32 1000 ("毫秒倍数")) -> ()  [unwired: 1 out]
            }
            frame #3 {
              w6070 = u8 0 items=["Normal", "Listen Only"] ("工作方式")
              w6071 = u8 1 items=["Dual Filter", "Single Filter"] ("滤波方式")
              n4212 = local read "设备索引号"() -> (w6075:u16)
              n4213 = local read "CAN卡类型"() -> (w6076:u32)
              n4214 = global write "EV05全局变量1.vi" "流控帧 2"(FALSE ("流控帧 2")) -> ()
              n4215 = local read "CAN端口"() -> (w6074:u16)
              n4216 = local write "控制1"(FALSE ("控制1")) -> ()
              n4217 = local write "消除"(FALSE ("消除")) -> ()
              n4218 = call "CAN_Init-8.6.vi"("CAN卡类型"=w6076, "设备索引号"=w6075, "CAN端口"=w6074, "操作类型"=enum16{"初始化CAN", "关闭CAN"}."初始化CAN", "滤波方式"=w6071, "Accept Code"=u32 3221225472, "簇"=T23 {"打开CAN"=FALSE, "初始化CAN"=TRUE, "开始CAN"=TRUE, "重启"=FALSE, "关闭CAN"=FALSE}, "Mask Code"=u32 1073741823 ("Accept Code"), "工作方式"=w6070, "是否滤波"=TRUE, "滤波选择"=T22 {"fiter_mode"=1, "fiter_endid"=402653184, "fiter_startid"=419430399}) -> ()  [unwired: 3 in, 6 out]
              n4219 = call <vilib>:"Unset Busy.vi"() -> ()  [unwired: 2 in, 10 out]
            }
          }
        }
        frame "强制均衡" {
          n4220 = local read "从板板号"() -> (w6080:u8)
          n4221 = stacked-sequence {
            tunnel: 133 -> [_ w6111 _ _]
            tunnel: w6080 -> [_ _ _ _]
            frame #0 {
              w6090 = u8 0 items=["Normal", "Listen Only"] ("工作方式")
              w6089 = u8 1 items=["Dual Filter", "Single Filter"] ("滤波方式")
              n4222 = global write "EV05全局变量1.vi" "读取超时"(FALSE ("读取超时")) -> ()
              n4223 = global write "EV05全局变量1.vi" "流控帧 2"(TRUE ("流控帧 2")) -> ()
              n4224 = local write "写?"(TRUE ("写?")) -> ()
              n4225 = local read "设备索引号"() -> (w6085:u16)
              n4226 = local read "CAN卡类型"() -> (w6084:u32)
              n4227 = local write "控制1"(TRUE ("控制1")) -> ()
              n4228 = local read "CAN端口"() -> (w6086:u16)
              n4229 = local write "消除"(TRUE ("消除")) -> ()
              n4230 = global write "EV05全局变量1.vi" "流控帧"(FALSE ("流控帧")) -> ()
              n4231 = call "CAN_Init-8.6.vi"("CAN卡类型"=w6084, "设备索引号"=w6085, "CAN端口"=w6086, "操作类型"=enum16{"初始化CAN", "关闭CAN"}."初始化CAN", "滤波方式"=w6089, "Accept Code"=u32 606601216, "簇"=T23 {"打开CAN"=FALSE, "初始化CAN"=TRUE, "开始CAN"=TRUE, "重启"=FALSE, "关闭CAN"=FALSE}, "Mask Code"=u32 524287 ("Accept Code"), "工作方式"=w6090, "是否滤波"=TRUE, "滤波选择"=T22 {"fiter_mode"=1, "fiter_endid"=75825152, "fiter_startid"=75890687}) -> ()  [unwired: 3 in, 6 out]
              n4232 = Wait Until Next ms Multiple(millisecond multiple=u32 20 ("毫秒倍数")) -> ()  [unwired: 1 out]
            }
            frame #1 {
              n4233 = local read "强制类型"() -> (w6117:enum16{"全通道开启", "单通道开启", "清待均衡时间"})
              n4234 = case shown="\"清待均衡时间\"" w6117 {
                tunnel: [250 252 254] -> w6107
                tunnel: [_ w6136 _] -> w6106
                tunnel: [_ w6135 _] -> w6105
                tunnel: [_ w6126 _] -> w6104
                tunnel: [_ w6119 _] -> w6103
                frame "全通道开启", Default {
                }
                frame "单通道开启" {
                  n4235 = local read "均衡类型选择"() -> (w6134:enum16{"放电均衡", "充电均衡", "充放电均衡"})
                  n4236 = local read "均衡位置"() -> (w6129:u16)
                  n4237 = case shown="\"放电均衡\", 默认" w6134 {
                    tunnel: [0 1] -> w6133
                    frame "放电均衡", Default {
                    }
                    frame "充电均衡" {
                    }
                  }
                  n4238 = Multiply(x="均衡时间", y=6.0) -> (x*y=w6121:dbl)
                  n4239 = Quotient & Remainder(x=w6121, y=256.0) -> (x-y*floor(x/y)=w6119:dbl, floor(x/y)=w6120:dbl)
                  n4240 = call "二进制解析-8.6.vi"("索引"=1, "数值"=w6133) -> ("低位子数组"=w6124:i32[])  [unwired: 1 in, 2 out]
                  n4241 = Quotient & Remainder(x=w6129, y=256.0) -> (x-y*floor(x/y)=w6135:dbl, floor(x/y)=w6136:dbl)
                  n4242 = call "二进制解析-8.6.vi"("索引"=8, "数值"=w6120) -> ("低位子数组"=w6125:i32[])  [unwired: 1 in, 2 out]
                  n4243 = Replace Array Subset(array=w6125, new element=w6124, index=0 ("索引")) -> (w6122:i32[])
                  n4244 = call "数值二进制转十进制-8.6.vi"("子数组"=w6122) -> ("十进制数值"=w6126:i32)  [unwired: 4 in]
                }
                frame "清待均衡时间" {
                }
              }
              n4245 = local write "命令"(w6111) -> ()
              n4246 = call "ID组合.vi"("SA(4)"=0 ("PDU(1)"), "PS(3)"=63 ("PDU(1)"), "PF(2)"=w6111, "PDU(1)"=4) -> ("ID"=w6110:i32)  [unwired: 7 out]
              n4247 = local read "设备索引号"() -> (w6114:u16)
              n4248 = local read "CAN卡类型"() -> (w6115:u32)
              n4249 = local read "CAN端口"() -> (w6113:u16)
              n4250 = local write "命令序号"(w6107) -> ()
              n4251 = Build Array(6, 4, w6107, w6106, w6105, w6104, w6103) -> (w6116:dbl[])
              n4252 = call "transmit-8.6.vi"("can卡类型"=w6115, "设备索引号"=w6114, "CAN端口"=w6113, "ID"=w6110, "SendType"=u8 0, "Data"=w6116) -> ()  [unwired: 3 in, 11 out]
            }
            frame #2 {
              n4253 = Wait Until Next ms Multiple(millisecond multiple=u32 1000 ("毫秒倍数")) -> ()  [unwired: 1 out]
            }
            frame #3 {
              w6150 = u8 0 items=["Normal", "Listen Only"] ("工作方式")
              w6149 = u8 1 items=["Dual Filter", "Single Filter"] ("滤波方式")
              n4254 = global write "EV05全局变量1.vi" "流控帧 2"(FALSE ("流控帧 2")) -> ()
              n4255 = local write "控制1"(FALSE ("控制1")) -> ()
              n4256 = local read "设备索引号"() -> (w6145:u16)
              n4257 = local read "CAN卡类型"() -> (w6144:u32)
              n4258 = local write "消除"(FALSE ("消除")) -> ()
              n4259 = local read "CAN端口"() -> (w6146:u16)
              n4260 = call <vilib>:"Unset Busy.vi"() -> ()  [unwired: 2 in, 10 out]
